vi "Actor Core.vi"(8 "error in":errorcluster, 11 "HVAC in":refnum<class "HVAC.lvclass">) -> (0 "error out":errorcluster, 3 "Actor out":refnum<class "Actor.lvclass">)   [LabVIEW 2018, in "HVAC Actor.lvlib" / "HVAC.lvclass"]
doc: "(<B>Filename</B>: Actor Framework.lvlib:Actor.lvclass:Actor Core.vi)\n\nReceives messages to the actor, reacts to them, and initiates any error handling that may shut the actor down.\n\nDescendant classes may override this VI to append parallel tasks for the actor to complete while it handles messages. Overrides use the Call Parent Method node."
uses:
  HVAC.lvclass
  C:/Users/Administrator/Desktop/2018LabVIEW EMS/EMS Generic Actor/EMS Generic/EMS Generic.lvclass
  <vilib>/ActorFramework/Actor/Actor.lvclass
  EMS Generic Actor/EMS Generic/EMS Generic.lvclass/EMS Generic.ctl
  <vilib>/ORNL/CSEISMIC DDS/CSEISMIC DDS Base/CSEISMIC DDS.lvclass/CSEISMIC DDS.ctl
  <vilib>/ORNL/CSEISMIC DDS/CSEISMIC DDS Base/Accessors/Write DDS Reference.vi
  <vilib>/ORNL/CSEISMIC DDS/CSEISMIC DDS Base/Accessors/Read DDS Reference.vi
  <vilib>/ORNL/CSEISMIC DDS/DDS Reader/DDS Reader.lvclass
  C:/Program Files (x86)/National Instruments/LabVIEW 2018/vi.lib/ORNL/CSEISMIC DDS/CSEISMIC DDS Base/CSEISMIC DDS.lvclass
  <vilib>/ORNL/CSEISMIC DDS/CSEISMIC DDS Base/Error Handler.vi
  Device DDS Communications Framework/Device DDS Communications/Device DDS Communications.lvclass
  EMS Generic Actor/EMS Generic/EMS Generic.lvclass
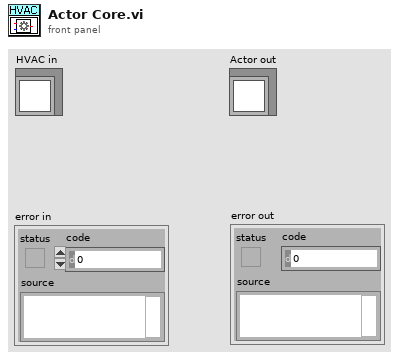
[diagram p1: front panel]
types:
  T1 = typedef "CSEISMIC DDS.lvlib/CSEISMIC DDS.lvclass/DeviceID.ctl" = string
  T2 = typedef "CSEISMIC DDS.lvlib/CSEISMIC DDS.lvclass/HVAC_Status.ctl" = cluster{"DeviceID":T1, "TemperatureSetpoint(degC)":dbl, "ControlMode":T3}
  T3 = typedef "CSEISMIC DDS.lvlib/CSEISMIC DDS.lvclass/ControlMode.ctl" = enum32{"Invalid", "Cooling", "Heating"}
  T4 = typedef "LVDDS_library.lvlib/DDS Sample Info.ctl" = cluster{"DDS_SampleStateKind":enum32{"DDS_INVALID_SAMPLE_STATE", "DDS_READ_SAMPLE_STATE", "DDS_NOT_READ_SAMPLE_STATE"}, "DDS_ViewStateKind":enum32{"DDS_INVALID_SAMPLE_STATE", "DDS_NEW_VIEW_STATE", "DDS_NOT_NEW_VIEW_STATE"}, "DDS_InstanceStateKind":enum32{"DDS_INVALID_STATE", "DDS_ALIVE_INSTANCE_STATE", "DDS_NOT_ALIVE_DISPOSED_INSTANCE_STATE", "", "DDS_NOT_ALIVE_NO_WRITERS_INSTANCE_STATE"}, "sec":i32, "nanosec":u32, "valid_data":bool}
  T5 = typedef "CSEISMIC DDS.lvlib/CSEISMIC DDS.lvclass/HVAC_Measurement.ctl" = cluster{"DeviceID":T1, "Temperature(degC)":dbl}
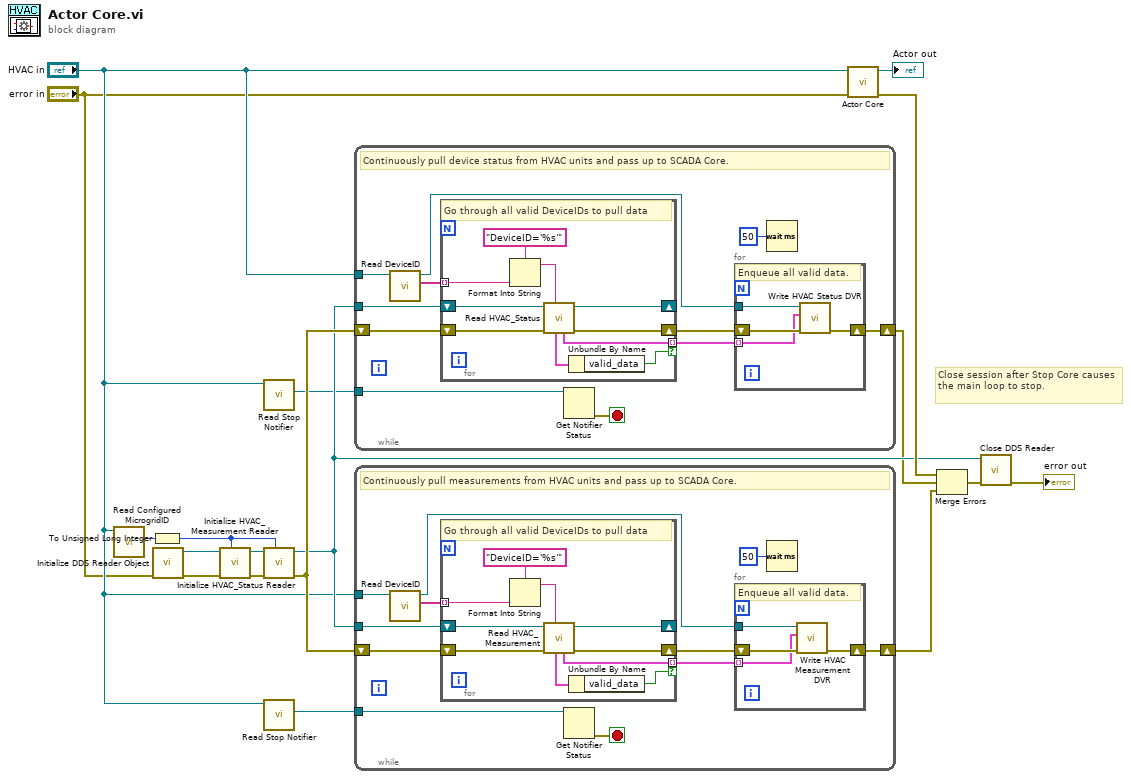
[diagram p0: block diagram]
diagram:
  # "Close session after Stop Core causes the main loop to stop."
  n1 = call "Read Configured MicrogridID.vi"("EMS Generic in"="HVAC in") -> ("Microgrid ID"=w18:u8)  [unwired: 8 in, 2 out]
  n2 = To Unsigned Long Integer(number=w18) -> (unsigned 32bit integer=w2:u32)
  n3 = call <vilib>:"Initialize DDS Reader Object.vi"("error in"="error in") -> ("error out"=w14:errorcluster, "DDS Reader out"=w13:refnum<class "DDS Reader.lvclass">)  [unwired: 9 in]
  n4 = call <vilib>:"Initialize HVAC_Measurement Reader.vi"("MicrogridID"=w2, "error in"=w14, "DDS Reader in"=w13) -> ("error out"=w15:errorcluster, "DDS Reader out"=w12:refnum<class "DDS Reader.lvclass">)  [unwired: 7 in]
  n5 = call "Read Stop Notifier.vi"("EMS Generic in"="HVAC in") -> ("stop"=w7:refnum<notifier>)  [unwired: 9 in, 1 out]
  n6 = call <vilib>:"Initialize HVAC_Status Reader.vi"("MicrogridID"=w2, "error in"=w15, "DDS Reader in"=w12) -> ("error out"=w11:errorcluster, "DDS Reader out"=w10:refnum<class "DDS Reader.lvclass">)  [unwired: 7 in]
  n7 = call "Read Stop Notifier.vi"("EMS Generic in"="HVAC in") -> ("stop"=w8:refnum<notifier>)  [unwired: 9 in, 1 out]
  n8 = while {
    tunnel: w7 -> [w29]
    shift-right: [w28] -> w5
    shift-left: w11 -> [w23]
    tunnel: "HVAC in" -> [w25]
    tunnel: w10 -> [w22]
    stop <- w27 stop-if-true
    # "Continuously pull device status from HVAC units and pass up to SCADA Core."
    n9 = call-dynamic "Read DeviceID.vi"("Device DDS Communications in"=w25) -> ("DeviceID"=w24:T1[], "Device DDS Communications out"=w19:refnum<class "HVAC.lvclass">)  [unwired: 9 in]
    n10 = for {
      shift-right: [w42] -> _
      shift-left: w22 -> [w43]
      shift-right: [w41] -> w21
      shift-left: w23 -> [w40]
      tunnel: w24 -> [w38] mode=indexing
      tunnel: [w35] -> w20 mode=indexing if=w34
      # "Go through all valid DeviceIDs to pull data"
      n11 = Format Into String(format string="DeviceID='%s'", w38) -> (resulting string=w37:string)  [unwired: 2 in, 1 out]
      n12 = call <vilib>:"Read HVAC_Status.vi"("Query condition"=w37, "error in"=w40, "DDS Reader in"=w43) -> ("error out"=w41:errorcluster, "DDS Reader out"=w42:refnum<class "DDS Reader.lvclass">, "data"=w35:T2, "DDS Sample Info"=w36:T4)  [unwired: 5 in]
      n13 = Unbundle By Name(w36) -> ("valid_data"=w34:bool)
    }
    n14 = Get Notifier Status(notifier=w29) -> (error out=w27:errorcluster)  [unwired: 1 in, 4 out]
    n15 = for {
      shift-right: [w32] -> w28
      shift-left: w21 -> [w33]
      tunnel: w20 -> [w31] mode=indexing
      tunnel: w19 -> [w30]
      # "Enqueue all valid data."
      n16 = call "Write HVAC Status DVR.vi"("error in"=w33, "HVAC_Status"=w31, "EMS Generic in"=w30) -> ("error out"=w32:errorcluster)  [unwired: 7 in, 1 out]
    }
    n17 = Wait (ms)(milliseconds to wait=u32 50) -> ()  [unwired: 1 out]
  }
  n18 = while {
    tunnel: w8 -> [w54]
    shift-right: [w53] -> w4
    shift-left: w11 -> [w48]
    tunnel: "HVAC in" -> [w50]
    tunnel: w10 -> [w47]
    stop <- w52 stop-if-true
    # "Continuously pull measurements from HVAC units and pass up to SCADA Core."
    n19 = call-dynamic "Read DeviceID.vi"("Device DDS Communications in"=w50) -> ("DeviceID"=w49:T1[], "Device DDS Communications out"=w44:refnum<class "HVAC.lvclass">)  [unwired: 9 in]
    n20 = for {
      shift-right: [w67] -> _
      shift-left: w47 -> [w68]
      shift-right: [w66] -> w46
      shift-left: w48 -> [w65]
      tunnel: w49 -> [w63] mode=indexing
      tunnel: [w60] -> w45 mode=indexing if=w59
      # "Go through all valid DeviceIDs to pull data"
      n21 = Format Into String(format string="DeviceID='%s'", w63) -> (resulting string=w62:string)  [unwired: 2 in, 1 out]
      n22 = call <vilib>:"Read HVAC_Measurement.vi"("Query condition"=w62, "error in"=w65, "DDS Reader in"=w68) -> ("error out"=w66:errorcluster, "DDS Reader out"=w67:refnum<class "DDS Reader.lvclass">, "data"=w60:T5, "DDS Sample Info"=w61:T4)  [unwired: 5 in]
      n23 = Unbundle By Name(w61) -> ("valid_data"=w59:bool)
    }
    n24 = Get Notifier Status(notifier=w54) -> (error out=w52:errorcluster)  [unwired: 1 in, 4 out]
    n25 = for {
      shift-right: [w57] -> w53
      shift-left: w46 -> [w58]
      tunnel: w45 -> [w56] mode=indexing
      tunnel: w44 -> [w55]
      # "Enqueue all valid data."
      n26 = call "Write HVAC Measurement DVR.vi"("error in"=w58, "HVAC_Measurement"=w56, "EMS Generic in"=w55) -> ("error out"=w57:errorcluster)  [unwired: 7 in, 1 out]
    }
    n27 = Wait (ms)(milliseconds to wait=u32 50) -> ()  [unwired: 1 out]
  }
  n28 = call-parent "Actor Core.vi"("error in"="error in", "Actor in"="HVAC in") -> ("error out"=w16:errorcluster, "Actor out"=→"Actor out":refnum<class "Actor.lvclass">)  [unwired: 8 in]
  n29 = Merge Errors(w16, w5, w4) -> (w6:errorcluster)
  n30 = call <vilib>:"Close DDS Reader.vi"("error in"=w6, "DDS Reader in"=w10) -> ("error out"=→"error out":errorcluster)  [unwired: 9 in]
